vi "Read Data.vi"(8 "error in (no error)":errorcluster, 10 "Read Size":i32, 11 "IntanElectrophysiology in":refnum<class "IntanElectrophysiology.lvclass">) -> (0 "error out":errorcluster, 2 "data":i32[][](array[numeric]), 3 "IntanElectrophysiology out":refnum<class "IntanElectrophysiology.lvclass">)   [LabVIEW 2014, in "IntanElectrophysiology.lvclass"]
uses:
  IntanElectrophysiology.lvclass
  IntanElectrophysiology.lvclass/IntanElectrophysiology.ctl
  AcquireTraces/AcquireTraces.lvclass/AcquireTraces.ctl
  AcquireTraces/AcquireTraces.lvclass
panel:
  in  "arg1":i16
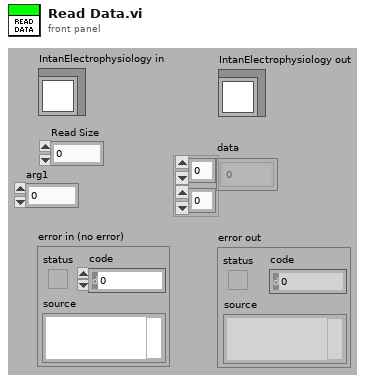
[diagram p1: front panel]
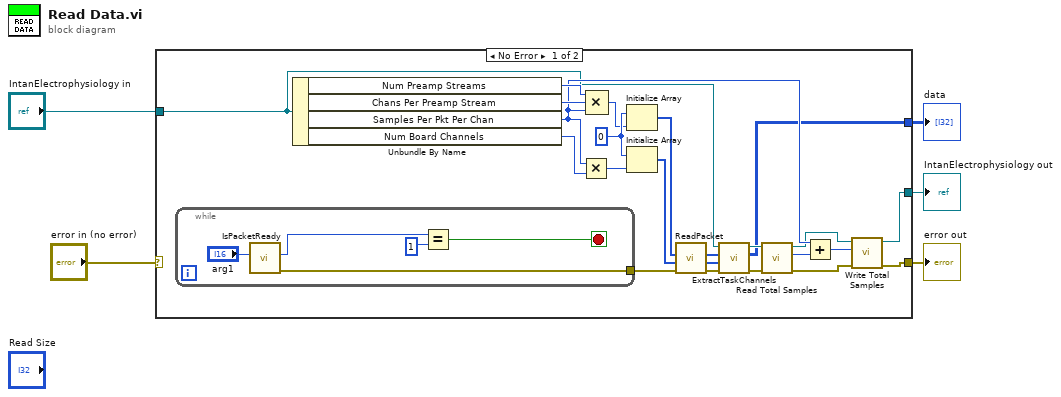
[diagram p0: block diagram]
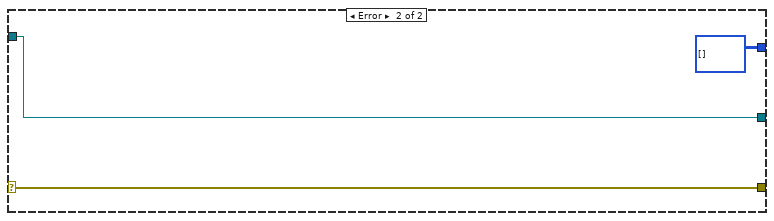
[diagram p2: hidden frame]
diagram:
  n1 = case shown="No Error" "error in (no error)" {
    selector: "error in (no error)" -> [_ w36]
    tunnel: [w17 w36] -> w2
    tunnel: [w16 w35] -> w3
    tunnel: "IntanElectrophysiology in" -> [w10 w35]
    tunnel: [w8 i32[][] [] ("data")] -> w5
    frame No Error {
      w25 = u32 0 ("element")
      n2 = while {
        tunnel: [w29] -> w28
        stop <- w30 stop-if-true
        n3 = call "IsPacketReady.vi"("arg1"="arg1") -> ("error out"=w29:errorcluster, "arg1 2"=w32:i16)  [unwired: 8 in, 1 out]
        n4 = Equal?(x=w32, y=i16 1) -> (x = y?=w30:bool)
      }
      n5 = Unbundle By Name(w10) -> ("Num Preamp Streams"=w27:i32, "Chans Per Preamp Stream"=w26:i32, "Samples Per Pkt Per Chan"=w19:i32, "Num Board Channels"=w23:i32)
      n6 = Multiply(x=w19, y=w23) -> (x*y=w22:i32)
      n7 = Compound Arithmetic op=MULTIPLY(w27, w26, w19) -> (w24:i32)
      n8 = Initialize Array(w25, w24) -> (w21:u32[])
      n9 = Initialize Array(w25, w22) -> (w20:u32[])
      n10 = call "ReadPacket.vi"("error in (no error)"=w28, "Board Array"=w20, "Preamp Array"=w21) -> ("error out"=w7:errorcluster, "Board Data"=w11:u16[], "Preamp Data"=w12:u16[])  [unwired: 5 in, 1 out]
      n11 = call "ExtractTaskChannels.vi"("error in (no error)"=w7, "Board Data"=w11, "Preamp Data"=w12, "IntanElectrophysiology in"=w10) -> ("error out"=w6:errorcluster, "Extracted Data"=w8:i32[][], "IntanElectrophysiology out"=w9:refnum<class "IntanElectrophysiology.lvclass">)  [unwired: 5 in]
      n12 = call-dynamic "Read Total Samples.vi"("error in (no error)"=w6, "AcquireTraces in"=w9) -> ("error out"=w13:errorcluster, "Total Samples"=w15:u64, "AcquireTraces out"=w14:refnum<class "IntanElectrophysiology.lvclass">)  [unwired: 7 in]
      n13 = Add(x=w19, y=w15) -> (x+y=w18:u64)
      n14 = call "Write Total Samples.vi"("error in (no error)"=w13, "Total Samples"=w18, "AcquireTraces in"=w14) -> ("error out"=w17:errorcluster, "AcquireTraces out"=w16:refnum<class "IntanElectrophysiology.lvclass">)  [unwired: 7 in]
    }
    frame Error {
    }
  }
  "error out" <- w2
  "IntanElectrophysiology out" <- w3
  "data" <- w5
